vi "GetDataSetRegistrations.vi"(8 "error in (no error)":errorcluster, 10 "data group name":string, 11 "virtual channel config":T1) -> (0 "error out":errorcluster, 1 "atleast one data set to register":bool, 2 "register data set":T3)   [LabVIEW 2017, in "CmsVirtualChannel.lvlib"]
uses:
  <vilib>/addons/InsightCM/Devices/Shared/Cms/CmsVirtualChannel/CmsVirtualChannel.lvlib
  <vilib>/addons/InsightCM/Devices/Shared/Common/DataEventCreator/controls/RegisterDataSets.ctl
  <vilib>/addons/InsightCM/Devices/Shared/Cms/CmsDataEventCreator/controls/DataSetRegistry.ctl
  <vilib>/addons/InsightCM/Devices/Shared/Common/DataEvent/controls/DataSetType.ctl
  <vilib>/addons/InsightCM/Devices/Shared/Cms/CmsVirtualChannel/controls/VirtualChannelGroup.ctl
  <vilib>/addons/InsightCM/Devices/Shared/Cms/CmsVirtualChannel/controls/VirtualChannel.ctl
  <vilib>/addons/InsightCM/Devices/Shared/Common/DataEvent/DataEvent.lvlib
  <vilib>/addons/InsightCM/Devices/Shared/Cms/CmsDataEventCreator/CmsDataEventCreator.lvlib
  <vilib>/addons/InsightCM/Devices/Shared/Common/DataEventCreator/DataEventCreator.lvlib
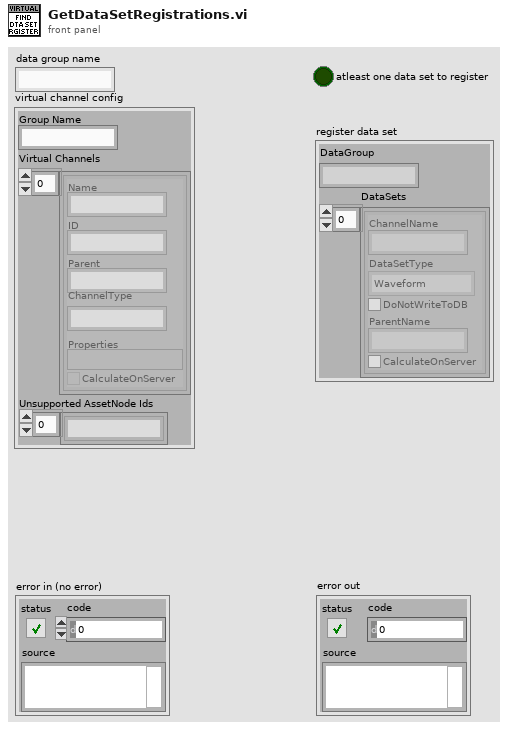
[diagram p1: front panel]
types:
  T1 = typedef "CmsVirtualChannel.lvlib/VirtualChannelGroup.ctl" = cluster{"Group Name":string, "Virtual Channels":T2[], "Unsupported AssetNode Ids":string[]}
  T2 = typedef "CmsVirtualChannel.lvlib/VirtualChannel.ctl" = cluster{"Name":string, "ID":string, "Parent":string, "ChannelType":string, "Properties":variant, "CalculateOnServer":bool}
  T3 = typedef "DataEventCreator.lvlib/RegisterDataSets.ctl" = cluster{"DataGroup":string, "DataSets":T4[]}
  T4 = typedef "CmsDataEventCreator.lvlib/DataSetRegistry.ctl" = cluster{"ChannelName":string, "DataSetType":T5, "DoNotWriteToDB":bool, "ParentName":string, "CalculateOnServer":bool}
  T5 = typedef "DataEvent.lvlib/DataSetType.ctl" = enum16{"Waveform", "SpeedProfile", "ThermalImage", "EmsaSweep"}
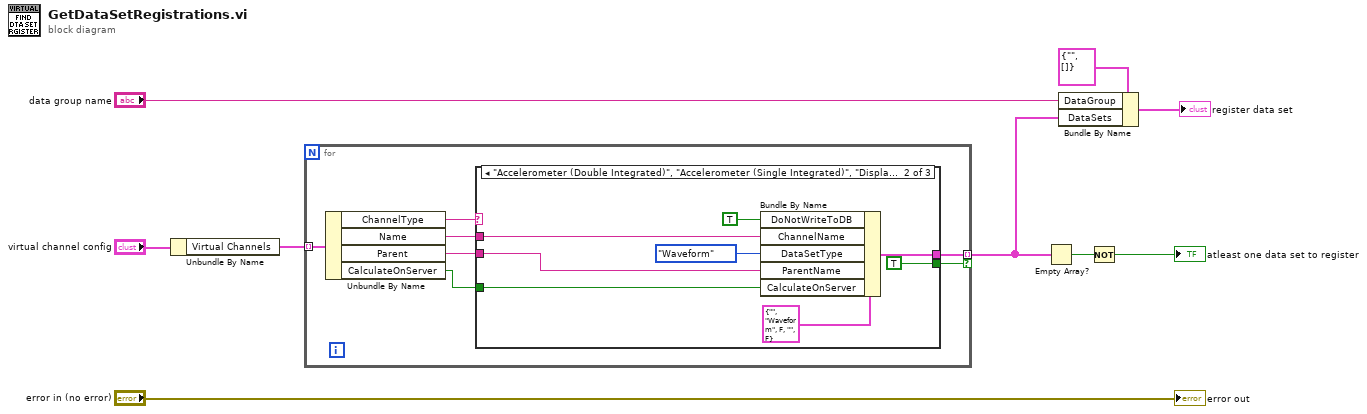
[diagram p0: block diagram]
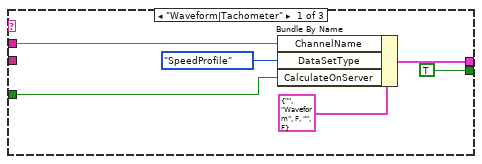
[diagram p2: hidden frame]
diagram:
  n1 = Unbundle By Name("virtual channel config") -> ("Virtual Channels"=w1:T2[])
  n2 = for {
    tunnel: [w16] -> w8 mode=indexing if=w15
    tunnel: w1 -> [w14] mode=indexing
    n3 = Unbundle By Name(w14) -> ("ChannelType"=w13:string, "Name"=w12:string, "Parent"=w11:string, "CalculateOnServer"=w10:bool)
    n4 = case shown="\"Accelerometer (Double Integrated)\", \"Accelerometer (Single Integrated)\", \"Displacement (Double Differentiated)\", \"Displacement (Single Differentiated)\", \"Velocity (Single Differentiated)\", \"Velocity (Single Integrated)\"" w13 {
      tunnel: w12 -> [w21 w29 _]
      tunnel: [w22 w30 _] -> w16
      tunnel: [TRUE TRUE _] -> w15
      tunnel: w11 -> [_ w24 _]
      tunnel: w10 -> [w17 w23 _]
      frame "Waveform|Tachometer" {
        n5 = Bundle By Name(cluster=T4 {"ChannelName"="", "DataSetType"=enum."Waveform", "DoNotWriteToDB"=FALSE, "ParentName"="", "CalculateOnServer"=FALSE} ("DataSet"), "ChannelName"=w21, "DataSetType"=DataSetType."SpeedProfile", "CalculateOnServer"=w17) -> (w22:T4)
      }
      frame "Accelerometer (Double Integrated)", "Accelerometer (Single Integrated)", "Displacement (Double Differentiated)", "Displacement (Single Differentiated)", "Velocity (Single Differentiated)", "Velocity (Single Integrated)" {
        n6 = Bundle By Name(cluster=T4 {"ChannelName"="", "DataSetType"=enum."Waveform", "DoNotWriteToDB"=FALSE, "ParentName"="", "CalculateOnServer"=FALSE} ("DataSet"), "DoNotWriteToDB"=TRUE, "ChannelName"=w29, "DataSetType"=DataSetType."Waveform", "ParentName"=w24, "CalculateOnServer"=w23) -> (w30:T4)
      }
      frame Default {
      }
    }
  }
  n7 = Empty Array?(array=w8) -> (empty?=w7:bool)
  n8 = Bundle By Name(cluster=T3 {"DataGroup"="", "DataSets"=[]} ("RegisterDataSet"), "DataGroup"="data group name", "DataSets"=w8) -> (→"register data set":T3)
  n9 = Not(x=w7) -> (.not. x?=→"atleast one data set to register":bool)
  "error out" <- "error in (no error)"
